vi "Read Device Identification.vi"(8 "error in":errorcluster, 9 "read device ID code":T2, 10 "object ID":u8, 11 "Modbus master in":refnum<class "Modbus Master.lvclass">) -> (0 "error out":errorcluster, 2 "objects":T1[](array[typedef]) {"Object ID" format="%x"}, 3 "Modbus master out":refnum<class "Modbus Master.lvclass">)   [LabVIEW 2015, in "Modbus Library.lvlib" / "Modbus Master.lvclass"]
doc: "Reads Modbus object information stored on the device. This can include basic information, like manufacturer, additional standard items, or model-specific extended items. This function may take a large amount of time to execute, as it requires the transfer of a large quantity of binary data. Even on TCP/IP, this function is limited by the maximum defined size of a Modbus protocol data unit."
uses:
  Modbus Master.lvclass
  Master Function Definition/Read Device ID code.ctl
  Data Model/Identification Parameters.ctl
  Modbus Master.lvclass/Modbus Master.ctl
  Modbus API.lvclass/Modbus API.ctl
  Transmission Data Unit/Transmission Data Unit.lvclass
  Data Model/Device Data Model.lvclass
  Modbus API.lvclass
  Master Function Definition/Master Function Definition.lvclass
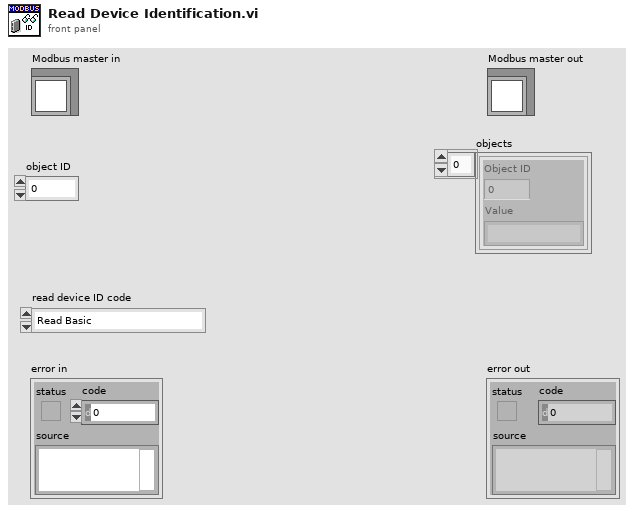
[diagram p1: front panel]
types:
  T1 = typedef "Modbus Library.lvlib/Device Data Model.lvclass/Identification Parameters.ctl" = cluster{"Object ID":u8, "Value":string}
  T2 = typedef "Modbus Library.lvlib/Device Data Model.lvclass/Read Device ID code.ctl" = enum8{"Read Basic", "Read Regular", "Read Extended", "Read Specific"}
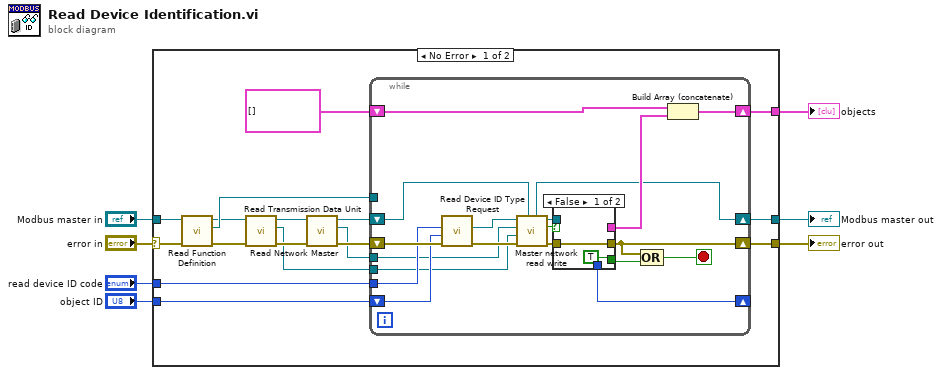
[diagram p0: block diagram]
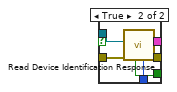
[diagram p2: hidden frame]
diagram:
  n1 = case shown="No Error" "error in" {
    selector: "error in" -> [w20 w53]
    tunnel: "Modbus master in" -> [w19 w52]
    tunnel: [w17 w52] -> w5
    tunnel: [w18 w53] -> w4
    tunnel: "read device ID code" -> [w24 _]
    tunnel: "object ID" -> [w23 _]
    tunnel: [w22 _] -> w1
    frame No Error {
      n2 = call "Read Function Definition.vi"("error in"=w20, "Modbus master in"=w19) -> ("error out"=w11:errorcluster, "master function definition"=w16:refnum<class "Master Function Definition.lvclass">, "Modbus master out"=w10:refnum<class "Modbus Master.lvclass">)  [unwired: 7 in]
      n3 = call "Read Transmission Data Unit.vi"("error in"=w11, "Modbus instance in"=w10) -> ("error out"=w12:errorcluster, "transmission data unit"=w9:refnum<class "Transmission Data Unit.lvclass">, "Modbus instance out"=w13:refnum<class "Modbus Master.lvclass">)  [unwired: 7 in]
      n4 = call "Read Network Master.vi"("error in"=w12, "Modbus master in"=w13) -> ("error out"=w15:errorcluster, "network master"=w8:refnum<class "Network Master.lvclass">, "Modbus master out"=w14:refnum<class "Modbus Master.lvclass">)  [unwired: 7 in]
      n5 = while {
        tunnel: w24 -> [w42]
        shift-right: [w39] -> w18
        shift-left: w15 -> [w43]
        shift-right: [w38] -> w22
        shift-left: T1[] [] -> [w37]
        shift-right: [w36] -> _
        shift-left: w23 -> [w41]
        shift-right: [w29] -> w17
        shift-left: w14 -> [w28]
        tunnel: w16 -> [_]
        tunnel: w9 -> [w27]
        tunnel: w8 -> [w26]
        stop <- w40 stop-if-true
        n6 = call "Read Device ID Type Request.vi"("error in"=w43, "Object ID"=w41, "Read Device ID Code"=w42) -> ("error out"=w30:errorcluster, "modbus data unit out"=w31:refnum<class "Modbus Data Unit.lvclass">)  [unwired: 7 in]
        n7 = call "Master network read write.vi"("Modbus master in"=w28, "error in"=w30, "transmission data unit in"=w27, "network master in"=w26, "Modbus data unit in"=w31) -> ("error out"=w33:errorcluster, "PDU Valid?"=w25:bool, "Modbus data unit out"=w32:refnum<class "Modbus Data Unit.lvclass">, "Modbus master out"=w29:refnum<class "Modbus Master.lvclass">)  [unwired: 3 in]
        n8 = case shown="False" w25 {
          tunnel: [w45 w51] -> w39
          tunnel: [_ w50] -> w36
          tunnel: [TRUE ("done?") w49] -> w35
          tunnel: [_ w48] -> w34
          tunnel: w33 -> [w45 w47]
          tunnel: w32 -> [_ w46]
          frame False {
          }
          frame True {
            n9 = call "Read Device Identification Response.vi"("error in"=w47, "modbus data unit in"=w46) -> ("error out"=w51:errorcluster, "Objects"=w48:T1[], "Next Object ID"=w50:u8, "done?"=w49:bool)  [unwired: 5 in, 1 out]
          }
        }
        n10 = Compound Arithmetic op=OR(w39, w35) -> (w40:bool)
        n11 = Build Array (concatenate)(w37, w34) -> (w38:T1[])
      }
    }
    frame Error {
    }
  }
  "error out" <- w4
  "Modbus master out" <- w5
  "objects" <- w1
